vi "UTILITY String to VISA.vi"(8 "error in (no error)":errorcluster, 11 "VISA Name":string) -> (0 "error out":errorcluster, 3 "VISA resource name out":refnum<visa-resource-name>)   [LabVIEW 2023]
uses:
  <vilib>/Instr/_visa.llb/VISA Find Search Mode.ctl
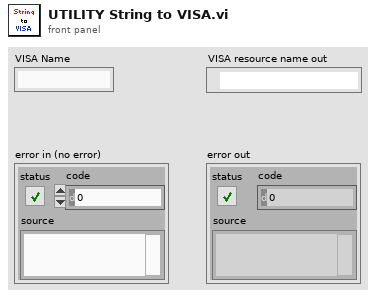
[diagram p1: front panel]
types:
  T1 = typedef "VISA Find Search Mode.ctl" = u32
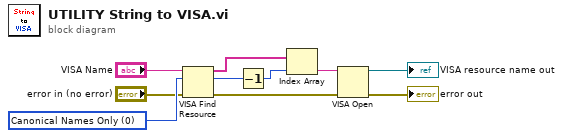
[diagram p0: block diagram]
diagram:
  w6 = T1 0 items=["Canonical Names Only"=0, "Aliases Only"=2, "Include Matching Aliases"=3, "Include All Aliases"=4] ("Search Mode")
  n1 = VISA Find Resource(8:"error in (no error)", 10:w6, 11:"VISA Name") -> (0:w2:errorcluster, 2:w8:u32, 3:w7:string[])
  n2 = Decrement(x=w8) -> (x-1=w9:u32)
  n3 = Index Array(array=w7, index=w9) -> (element=w10:string)
  n4 = VISA Open(error in (no error)=w2, VISA resource name=w10) -> (VISA resource name=→"VISA resource name out":refnum<visa-resource-name>, error out=→"error out":errorcluster)  [unwired: 3 in]
